vi "Init.vi"(10 "RefStringIn":refnum<vi>, 11 "Token":string) -> (2 "GlobalDataRef":refnum<data-value>, 3 "Queues":T1)   [LabVIEW 2015]
uses:
  Telegram/Methods/TypeDefs/Message.ctl
  TypeDefs/GlobalData.ctl
  Telegram/Methods/TypeDefs/ReplyKeyboardMarkup.ctl
  <vilib>/FPGAPlugInAG/myRIO-1900/niLvFpga_Open_myRIO-1900.vi
  <vilib>/rvi/interface/common/dynamic/niFpgaDynamicAddResources.vi
  <vilib>/rvi/interface/nirviOpenFPGA/nirviOpenFPGA.xnode
  FPGABitfiles/TelegramBot_FPGATarget_TopLevel_054DY+20zVc.lvbitx
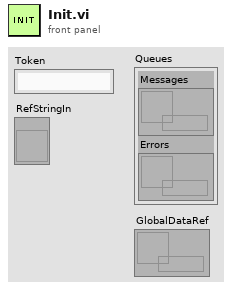
[diagram p1: front panel]
types:
  T1 = cluster{"Messages":refnum<queue>, "Errors":refnum<queue>}
  T2 = cluster{"Period":u32, "DutyCycle":u32, "Combo Box":string}[]
  T3 = typedef "GlobalData.ctl" = cluster{"FPGA VI Ref":refnum<k20>, "Token":string, "ActiveChats":cluster{"ChatId":i32, "Type":string}[], "ActiveKeyboards":cluster{"Chat#":i32, "ReplyKeyboardMarkup":T4}[], "RefStringIn":refnum<vi>}
  T4 = typedef "ReplyKeyboardMarkup.ctl" = cluster{"keyboard":cluster{"text":string, "req_loc":bool}[][], "resize_keyboard":bool, "one_time_keyboard":bool, "selective":bool}
  T5 = typedef "Message.ctl" = cluster{"update_id":u32, "from":string, "text":string, "date":timestamp, "chat_id":i32, "type":string, "reply_to_message.text":string, "message_id":u32}
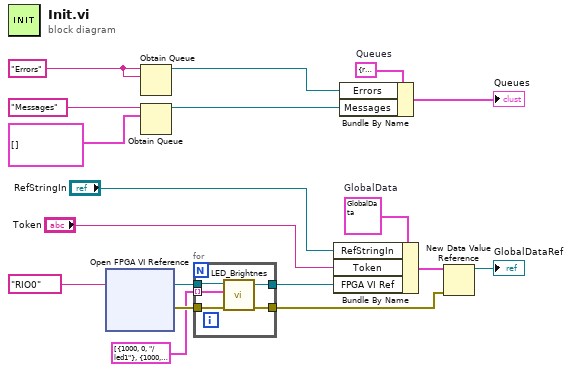
[diagram p0: block diagram]
diagram:
  w16 = T3 {"FPGA VI Ref"=refnum, "Token"="bot277787689:AAHmg4xfDwkElXKcgoITf0nrYVpOVlTc8k0/", "ActiveChats"=[], "ActiveKeyboards"=[], "RefStringIn"=refnum}  # GlobalData
  w13 = T1 {"Messages"=refnum, "Errors"=refnum}  # Queues
  w11 = "Errors" ("name (unnamed)")
  n1 = xnode "Open FPGA VI Reference"("resource name"=tag "RIO0") -> ("FPGA VI Reference Out"=w7:refnum<k20>, "error out"=w6:errorcluster)  [unwired: 1 in]
  n2 = Obtain Queue(name (unnamed)=w11, element data type=w11) -> (queue out=w8:refnum<queue>)  [unwired: 3 in, 2 out]
  n3 = Obtain Queue(name (unnamed)="Messages", element data type=T5[] [] ("Messages")) -> (queue out=w14:refnum<queue>)  [unwired: 3 in, 2 out]
  n4 = for {
    tunnel: w7 -> [w23]
    tunnel: [w22] -> w4
    tunnel: w6 -> [w21]
    tunnel: [w20] -> w3
    tunnel: T2 [{"Period"=1000, "DutyCycle"=0, "Combo Box"="/led1"}, {"Period"=1000, "DutyCycle"=0, "Combo Box"="/led2"}, {"Period"=1000, "DutyCycle"=0, "Combo Box"="/led3"}] -> [w19] mode=indexing
    n5 = call "LED_Brightnes.vi"("error in (no error)"=w21, "LEDParam"=w19, "FPGA VI"=w23) -> ("error out"=w20:errorcluster, "FPGA VI Reference Out"=w22:refnum<k20>)  [unwired: 7 in]
  }
  n6 = Bundle By Name(cluster=w16, "RefStringIn"="RefStringIn", "Token"="Token", "FPGA VI Ref"=w4) -> (w17:T3)
  n7 = Bundle By Name(cluster=w13, "Errors"=w8, "Messages"=w14) -> (→"Queues":T1)
  n8 = New Data Value Reference(data value=w17, error in=w3) -> (data value reference=→"GlobalDataRef":refnum<data-value>)  [unwired: 1 out]
